vi "Build Selected Item Tree.vi"(10 "Selections":i32[](array[numeric]), 11 "Items In":T1[](array[typedef])) -> (2 "Sorted Code Items":i32[](array[numeric]), 3 "Items":T1[](array[typedef]))   [LabVIEW 2020, in "TypeGraph.lvlib"]
uses:
  TypeGraph.lvlib
  Type Reflection Item.ctl
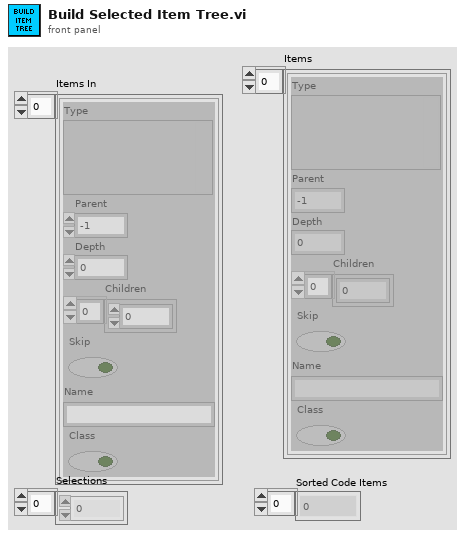
[diagram p1: front panel]
types:
  T1 = typedef "TypeGraph.lvlib/Type Reflection Item.ctl" = cluster{"Type":variant, "Parent":i32, "Depth":i32, "Children":i32[], "Skip":bool, "Name":string, "Class":bool}
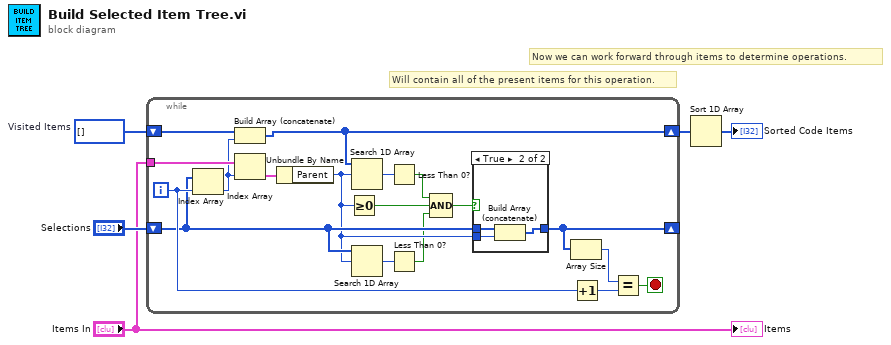
[diagram p0: block diagram]
diagram:
  w5 = i32[] []  # Visited Items
  # "Now we can work forward through items to determine operations."
  # "Will contain all of the present items for this operation."
  n1 = while {
    shift-right: [w17] -> w3
    shift-left: w5 -> [w22]
    tunnel: "Items In" -> [w23]
    shift-right: [w16] -> _
    shift-left: "Selections" -> [w8]
    i -> [w14]
    stop <- w15 stop-if-true
    n2 = Index Array(array=w8, index=w14) -> (element=w21:i32)
    n3 = Build Array (concatenate)(w22, w21) -> (w17:i32[])
    n4 = Index Array(array=w23, index=w21) -> (element=w20:T1)
    n5 = Unbundle By Name(w20) -> ("Parent"=w7:i32)
    n6 = Greater Or Equal To 0?(x=w7) -> (x >= 0?=w10:bool)
    n7 = Search 1D Array(1D array=w17, element=w7) -> (index of element=w19:i32)  [unwired: 1 in]
    n8 = Search 1D Array(1D array=w8, element=w7) -> (index of element=w9:i32)  [unwired: 1 in]
    n9 = Less Than 0?(x=w19) -> (x < 0?=w18:bool)
    n10 = Less Than 0?(x=w9) -> (x < 0?=w6:bool)
    n11 = Compound Arithmetic op=AND(w18, w10, w6) -> (w11:bool)
    n12 = case shown="True" w11 {
      tunnel: w8 -> [w24 w27]
      tunnel: w7 -> [_ w26]
      tunnel: [w24 w25] -> w16
      frame False {
      }
      frame True {
        n13 = Build Array (concatenate)(w27, w26) -> (w25:i32[])
      }
    }
    n14 = Array Size(array=w16) -> (size(s)=w13:i32)
    n15 = Increment(x=w14) -> (x+1=w12:i32)
    n16 = Equal?(x=w13, y=w12) -> (x = y?=w15:bool)
  }
  n17 = Sort 1D Array(array=w3) -> (sorted array=→"Sorted Code Items":i32[])
  "Items" <- "Items In"
